vi "AddParameters.vi"(0 "Automation Refnum in":refnum<k7>, 5 "Parameter Value Expression":string[](array[string]), 11 "Error In":errorcluster) -> (15 "Error Out":errorcluster)   [LabVIEW 2021, in "Create Sequence.lvlib"]
uses:
  Create Sequence.lvlib
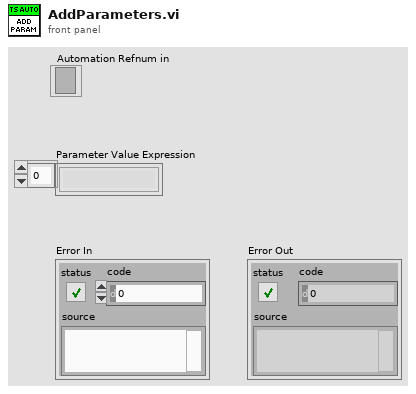
[diagram p1: front panel]
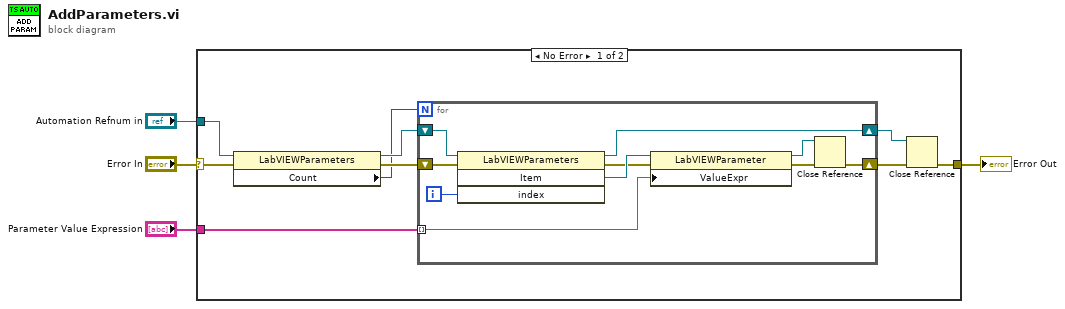
[diagram p0: block diagram]
diagram:
  n1 = case shown="No Error" "Error In" {
    selector: "Error In" -> [w10 w24]
    tunnel: [w13 w24] -> w4
    tunnel: "Automation Refnum in" -> [w8 _]
    tunnel: "Parameter Value Expression" -> [w5 _]
    frame No Error {
      n2 = property class="LabVIEWParameters"(reference=w8, error in=w10) -> (reference out=w11:refnum<k7>, error out=w12:errorcluster, "Count"=w9:i32)
      n3 = for {
        N: w9 -> [_]
        shift-right: [w21] -> w6
        shift-left: w11 -> [w23]
        shift-right: [w18] -> w7
        shift-left: w12 -> [w17]
        tunnel: w5 -> [w16] mode=indexing
        i -> [w15]
        n4 = invoke class="LabVIEWParameters" method="Item"(reference=w23, error in=w17, "index"=w15) -> (reference out=w21:refnum<k7>, error out=w14:errorcluster, "Item"=w22:refnum<k7>)  [unwired: 1 in, 1 out]
        n5 = property class="LabVIEWParameter"(reference=w22, error in=w14, "ValueExpr"=w16) -> (reference out=w20:refnum<k7>, error out=w19:errorcluster)
        n6 = Close Reference(reference=w20, error in (no error)=w19) -> (error out=w18:errorcluster)
      }
      n7 = Close Reference(reference=w6, error in (no error)=w7) -> (error out=w13:errorcluster)
    }
    frame Error {
    }
  }
  "Error Out" <- w4
